vi "Splashy.TestLauncher.vi"() -> ()   [LabVIEW 2020, in "Splashy.lvclass"]
doc: "JKI State Machine Objects (SMO) 1.0.0.5\nJKI - JKI\nCopyright (c) 2016, JKI"
uses:
  Splashy.lvclass
  C:/Program Files (x86)/National Instruments/LabVIEW 2020/vi.lib/JKI/JKI SMO/SMO/SMO.lvclass
  C:/Program Files (x86)/National Instruments/LabVIEW 2020/vi.lib/JKI/JKI SMO/SMO.UI/SMO.UI.lvclass
  <vilib>/JKI/JKI SMO/SMO/Typedefs/SMOState --Enum.ctl
  <vilib>/JKI/JKI SMO/SMO/SMO.lvclass
  <vilib>/JKI/JKI SMO/SMO.UI/SMO.UI.lvclass
panel:
  out "error out":errorcluster
  in  "Stop":bool
  # "SMO Splash Test Launcher"
  # "For instructions on how to use the JKI State Machine Objects, examples and video tutorials, visit:\nhttp://jki.net/state-machine-objects/\n\nJKI State Machine Objects™\nhttp://jki.net/state-machine-objects/\nCopyright (C) 2005-2015, JKI <info@jki.net>\nALL RIGHTS RESERVED"
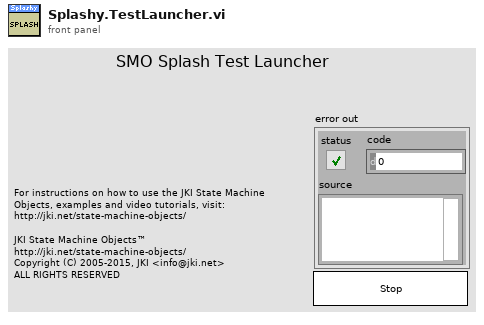
[diagram p1: front panel]
types:
  T1 = typedef "SMO.lvclass/Public Events.ctl" = cluster{"Error":refnum<user-event>, "State":refnum<user-event>, "Reserve State":refnum<user-event>}
  T2 = typedef "SMO.UI.lvclass/PublicEvents--Cluster.ctl" = cluster{"UI Hidden":refnum<user-event>, "UI State":refnum<user-event>}
  T3 = typedef "SMO.lvclass/SMOState --Enum.ctl" = enum16{"unknown", "Created", "Started", "Stopped"}
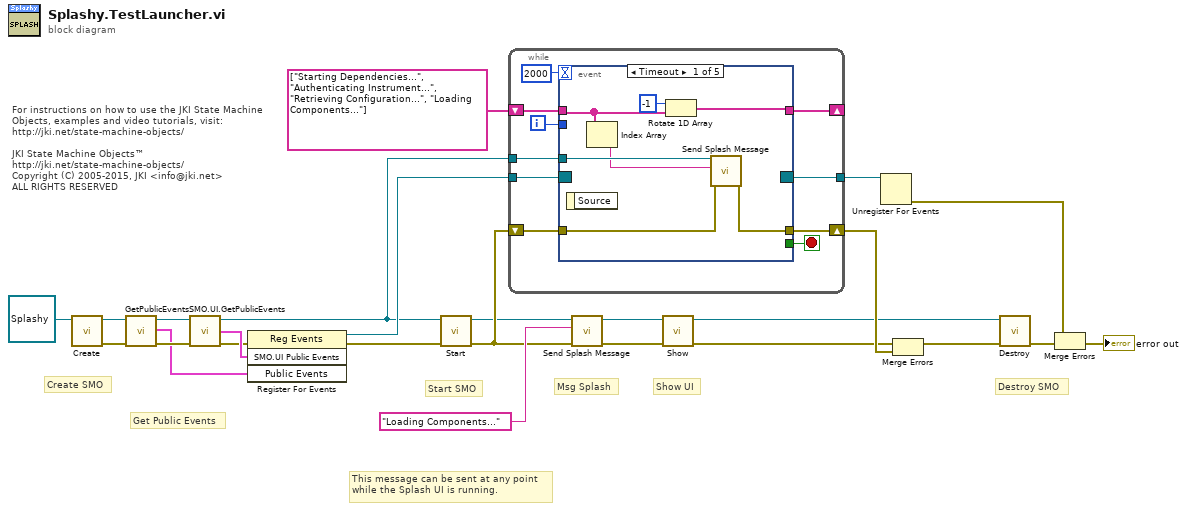
[diagram p0: block diagram]
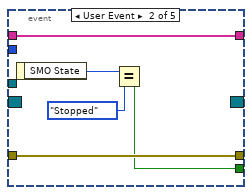
[diagram p2: hidden frame]
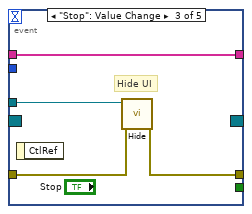
[diagram p3: hidden frame]
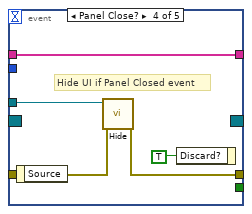
[diagram p4: hidden frame]
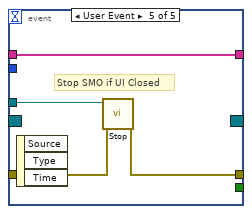
[diagram p5: hidden frame]
diagram:
  # "Msg Splash"
  # "This message can be sent at any point\nwhile the Splash UI is running."
  # "Show UI"
  # "For instructions on how to use the JKI State Machine Objects, examples and video tutorials, visit:\nhttp://jki.net/state-machine-objects/\n\nJKI State Machine Objects™\nhttp://jki.net/state-machine-objects/\nCopyright (C) 2005-2015, JKI <info@jki.net>\nALL RIGHTS RESERVED"
  # "Get Public Events"
  # "Start SMO"
  # "Destroy SMO"
  # "Create SMO"
  n1 = call <vilib>:"Create.vi"("SMO"=refnum<class "Splashy.lvclass"> refnum ("SMO.Template.lvclass")) -> ("error out"=w6:errorcluster, "SMO out"=w8:refnum<class "Splashy.lvclass">)  [unwired: 8 in, 1 out]
  n2 = call <vilib>:"GetPublicEvents.vi"("error in (no error)"=w6, "SMO"=w8) -> ("error out"=w5:errorcluster, "Public Events"=w4:T1, "SMO out"=w7:refnum<class "Splashy.lvclass">)  [unwired: 7 in]
  n3 = call <vilib>:"SMO.UI.GetPublicEvents.vi"("error in (no error)"=w5, "SMO.UI"=w7) -> ("error out"=w10:errorcluster, "SMO.UI Public Events"=w11:T2, "SMO.UI out"=w2:refnum<class "Splashy.lvclass">)  [unwired: 7 in]
  n4 = register-events(error in=w10, w11, w4) -> (reference out=w3:refnum<event-registration>, error out=w9:errorcluster)  [unwired: 1 in]
  n5 = call <vilib>:"Start.vi"("error in (no error)"=w9, "SMO"=w2) -> ("error out"=w15:errorcluster, "SMO out"=w12:refnum<class "Splashy.lvclass">)  [unwired: 8 in]
  n6 = while {
    shift-right: [w34] -> w24
    shift-left: w15 -> [w33]
    tunnel: w3 -> [w32]
    tunnel: [w31] -> w25
    tunnel: w2 -> [w30]
    shift-right: [w26] -> _
    shift-left: string[] ["Starting Dependencies...", "Authenticating Instrument...", "Retrieving Configuration...", "Loading Components..."] -> [w27]
    i -> [w28]
    stop <- w35 stop-if-true
    n7 = event shown="[0] Timeout" {
      selector: w32 -> [_ _ _ _ _]
      dyn-events: [_ _ _ _ _] -> w31
      timeout: 2000 -> [_ _ _ _ _]
      tunnel: [_ w44 _ _ _] -> w35
      tunnel: w30 -> [w42 _ w51 w55 w60]
      tunnel: [w39 w47 w49 w53 w59] -> w34
      tunnel: w33 -> [w40 w47 w50 w54 w58]
      tunnel: w28 -> [_ _ _ _ _]
      tunnel: w27 -> [w38 w43 w48 w52 w57]
      tunnel: [w37 w43 w48 w52 w57] -> w26
      event Timeout {
        n8 = event-data() -> ()  [unwired: 1 in, 1 out]
        n9 = Index Array(array=w38) -> (element=w41:string)  [unwired: 1 in]
        n10 = Rotate 1D Array(1:w38, 2:-1 ("n")) -> (0:w37:string[])
        n11 = call-dynamic "Send Splash Message.vi"("error in (no error)"=w40, "Message"=w41, "Splashy"=w42) -> ("error out"=w39:errorcluster)  [unwired: 7 in, 1 out]
      }
      event User Event {
        n12 = event-data() -> ("SMO State"=w46:T3)  [unwired: 1 in]
        n13 = Equal?(x=w46, y=SMOState_--Enum."Stopped") -> (x = y?=w44:bool)
      }
      event "Stop": Value Change {
        # "Hide UI"
        n14 = event-data() -> ()  [unwired: 1 in, 1 out]
        n15 = call <vilib>:"Hide.vi"("error in (no error)"=w50, "SMO.UI"=w51) -> ("error out"=w49:errorcluster)  [unwired: 8 in, 1 out]
      }
      event Panel Close? {
        # "Hide UI if Panel Closed event"
        n16 = event-data() -> ()  [unwired: 1 in, 1 out]
        n17 = call <vilib>:"Hide.vi"("error in (no error)"=w54, "SMO.UI"=w55) -> ("error out"=w53:errorcluster)  [unwired: 8 in, 1 out]
        n18 = event-data("Discard?"=TRUE ("OK")) -> ()  [unwired: 1 in, 1 out]
      }
      event User Event {
        # "Stop SMO if UI Closed"
        n19 = event-data() -> ()  [unwired: 1 in, 3 out]
        n20 = call <vilib>:"Stop.vi"("error in (no error)"=w58, "SMO"=w60) -> ("error out"=w59:errorcluster)  [unwired: 8 in, 1 out]
      }
    }
  }
  n21 = call-dynamic "Send Splash Message.vi"("error in (no error)"=w15, "Message"="Loading Components...", "Splashy"=w12) -> ("error out"=w14:errorcluster, "Splashy out"=w13:refnum<class "Splashy.lvclass">)  [unwired: 7 in]
  n22 = call <vilib>:"Show.vi"("error in (no error)"=w14, "SMO.UI"=w13) -> ("error out"=w19:errorcluster, "SMO.UI out"=w18:refnum<class "Splashy.lvclass">)  [unwired: 8 in]
  n23 = Unregister For Events(event registration refnum=w25) -> (error out=w23:errorcluster)  [unwired: 1 in]
  n24 = Merge Errors(w19, w24) -> (w17:errorcluster)
  n25 = call <vilib>:"Destroy.vi"("error in (no error)"=w17, "SMO"=w18) -> ("error out"=w21:errorcluster)  [unwired: 9 in]
  n26 = Merge Errors(w23, w21) -> (→"error out":errorcluster)
